vi "SVG2VSDX.vi"() -> ()   [LabVIEW 2018]
uses:
  <userlib>/_OpenG.lib/file/file.llb/Convert File Extension (Path)__ogtk.vi
panel:
  in  "使用源路径":bool=TRUE
  in  "Viso格式":enum32{"VSD", "VSDX"}(radio)=enum."VSDX"
  in  "Viso路径":path
  in  "SVG路径":path
  in  "转换":bool
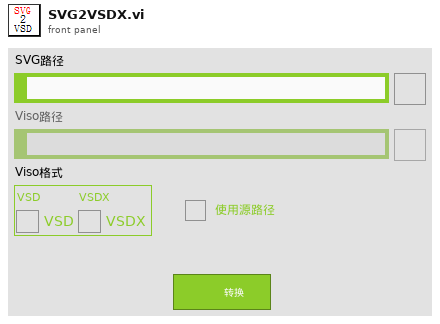
[diagram p1: front panel]
types:
  T1 = enum8{"Enabled", "Disabled", "Disabled and Grayed Out"}
  T2 = enum16{"Null", "NonExist", "EmptyFile", "File", "EmptyDir", "Directory"}
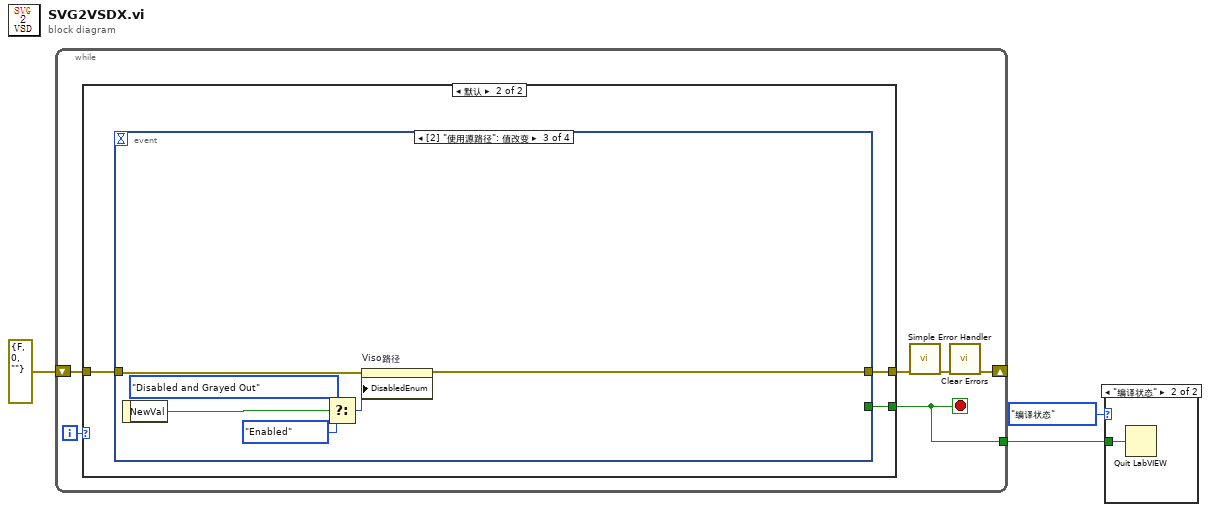
[diagram p0: block diagram]
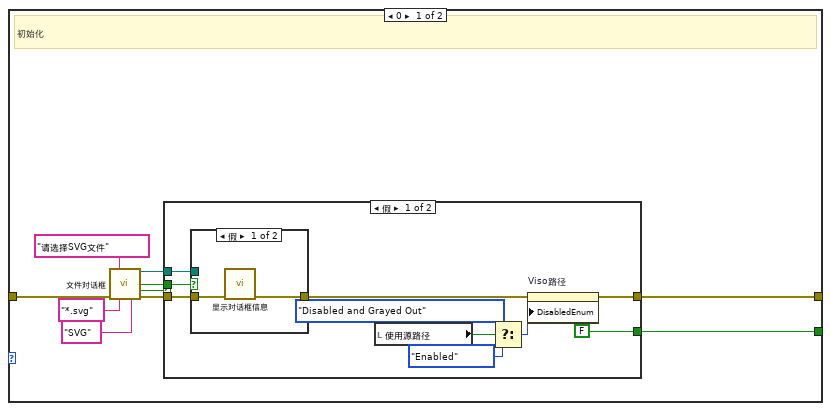
[diagram p3: hidden frame]
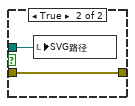
[diagram p4: hidden frame]
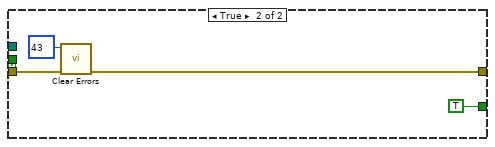
[diagram p5: hidden frame]
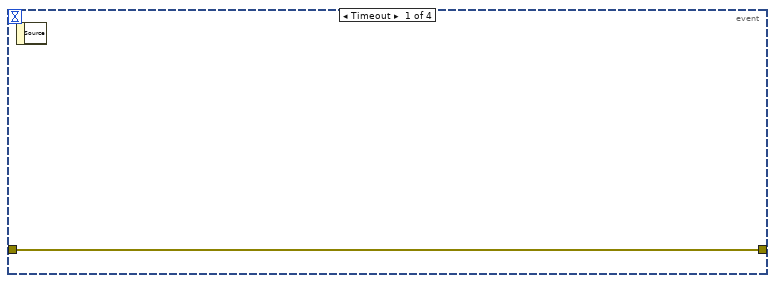
[diagram p6: hidden frame]
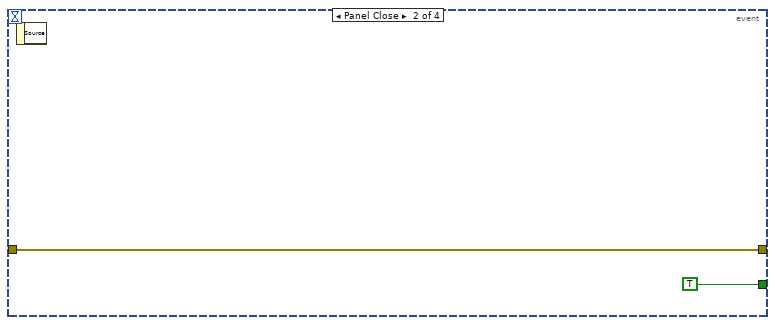
[diagram p7: hidden frame]
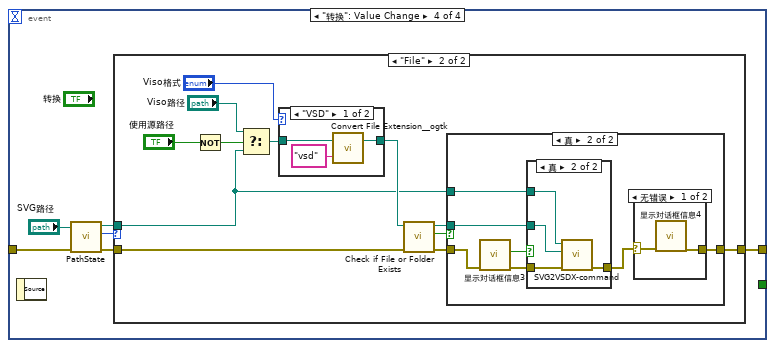
[diagram p8: hidden frame]
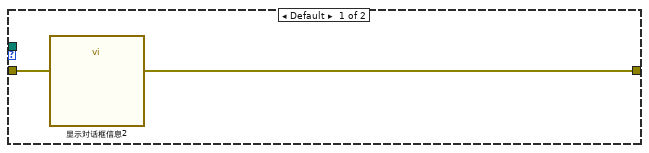
[diagram p9: hidden frame]
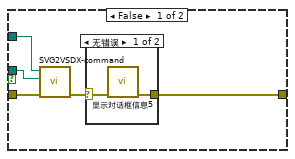
[diagram p10: hidden frame]
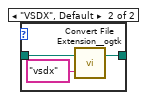
[diagram p14: hidden frame]
diagram:
  n1 = while {
    tunnel: [w4] -> w1
    shift-right: [w5] -> _
    shift-left: errorcluster {"status"=FALSE, "code"=0, "source"=""} ("Error in") -> [w8]
    i -> [w9]
    stop <- w4 stop-if-true
    n2 = case shown="默认" w9 {
      tunnel: w8 -> [w19 w40]
      tunnel: [w10 w39] -> w7
      tunnel: [w13 w38] -> w4
      frame 0 {
        # "初始化"
        n3 = call "文件对话框"("prompt"="请选择SVG文件", "error in"=w19, "pattern (all files)"="*.svg", "pattern label"="SVG") -> ("selected path"=w11:path, "exists"=w12:bool, "cancelled"=w14:bool, "error out"=w18:errorcluster)  [unwired: 8 in]
        n4 = case shown="假" w14 {
          tunnel: w18 -> [w29 w37]
          tunnel: [w25 w36] -> w10
          tunnel: [FALSE TRUE] -> w13
          tunnel: w12 -> [w27 _]
          tunnel: w11 -> [w26 _]
          frame False {
            n5 = case shown="假" w27 {
              tunnel: w29 -> [w31 w33]
              tunnel: [w30 w33] -> w24
              tunnel: w26 -> [_ w32]
              frame False {
                n6 = call "显示对话框信息"("error in (no error)"=w31) -> ("error out"=w30:errorcluster)  [unwired: 9 in, 1 out]
              }
              frame True {
                n7 = local write "SVG路径"(w32) -> ()
              }
            }
            n8 = local read "使用源路径"() -> (w20:bool)
            n9 = Select(t=T1."Disabled and Grayed Out" ("禁用"), s=w20, f=T1."Enabled" ("禁用")) -> (s? t:f=w21:T1)
            n10 = property on="Viso路径" class="Path"(error in=w24, "DisabledEnum"=w21) -> (error out=w25:errorcluster)  [unwired: 1 in, 1 out]
          }
          frame True {
            n11 = call <vilib>:"Clear Errors.vi"("error in (no error)"=w37, "specific error code to clear (0: all)"=43) -> ("error out"=w36:errorcluster)  [unwired: 4 in, 1 out]
          }
        }
      }
      frame Default {
        n12 = event shown="[2] \"使用源路径\": 值改变" {
          selector: _ -> [_ _ _ _]
          dyn-events: _ -> [_ _ _ _]
          timeout: _ -> [_ _ _ _]
          tunnel: w40 -> [w41 w43 w45 w55]
          tunnel: [w41 w43 w46 w52] -> w39
          tunnel: [_ TRUE _ _] -> w38
          event Timeout {
            n13 = event-data() -> ()  [unwired: 1 in, 1 out]
          }
          event Panel Close {
            n14 = event-data() -> ()  [unwired: 1 in, 1 out]
          }
          event "使用源路径": Value Change {
            n15 = event-data() -> ("NewVal"=w44:bool)  [unwired: 1 in]
            n16 = Select(t=T1."Disabled and Grayed Out" ("禁用"), s=w44, f=T1."Enabled" ("禁用")) -> (s? t:f=w47:T1)
            n17 = property on="Viso路径" class="Path"(error in=w45, "DisabledEnum"=w47) -> (error out=w46:errorcluster)  [unwired: 1 in, 1 out]
          }
          event "转换": Value Change {
            n18 = event-data() -> ()  [unwired: 1 in, 1 out]
            n19 = call <vilib>:"PathState.vi"("error in (no error)"=w55, "Path_input"="SVG路径") -> ("error out"=w54:errorcluster, "State"=w51:T2, "Path_output"=w50:path)  [unwired: 7 in]
            n20 = case shown="\"File\"" w51 {
              tunnel: w54 -> [w57 w69]
              tunnel: [w56 w63] -> w52
              tunnel: w50 -> [_ w58]
              frame Default {
                n21 = call "显示对话框信息2"("error in (no error)"=w57) -> ("error out"=w56:errorcluster)  [unwired: 9 in, 1 out]
              }
              frame "File" {
                n22 = Not(x="使用源路径") -> (.not. x?=w66:bool)
                n23 = Select(t="Viso路径", s=w66, f=w58) -> (s? t:f=w64:path)
                n24 = case shown="\"VSD\"" "Viso格式" {
                  tunnel: w64 -> [w95 w98]
                  tunnel: [w93 w96] -> w60
                  frame "VSD" {
                    n25 = call-poly <userlib>:"Convert File Extension__ogtk.vi"("new ending (none)"="vsd", "file name"=w95) -> ("new filename"=w93:path)  [unwired: 1 out]
                  }
                  frame "VSDX", Default {
                    n26 = call-poly <userlib>:"Convert File Extension__ogtk.vi"("new ending (none)"="vsdx", "file name"=w98) -> ("new filename"=w96:path)  [unwired: 1 out]
                  }
                }
                n27 = call <vilib>:"Check if File or Folder Exists.vi"("error in (no error)"=w69, "path"=w60) -> ("error out"=w62:errorcluster, "file or folder exists?"=w61:bool, "dup path"=w59:path)  [unwired: 7 in]
                n28 = case shown="真" w61 {
                  tunnel: w62 -> [w74 w84]
                  tunnel: [w71 w79] -> w63
                  tunnel: w59 -> [w72 w81]
                  tunnel: w58 -> [w73 w80]
                  frame False {
                    n29 = call "SVG2VSDX-command.vi"("Error in"=w74, "vsd路径"=w72, "svg路径"=w73) -> ("Error out"=w70:errorcluster)  [unwired: 8 in]
                    n30 = case shown="无错误" w70 {
                      selector: w70 -> [w75 w77]
                      tunnel: [w76 w77] -> w71
                      frame No Error {
                        n31 = call "显示对话框信息5"("error in (no error)"=w75) -> ("error out"=w76:errorcluster)  [unwired: 9 in, 1 out]
                      }
                      frame Error {
                      }
                    }
                  }
                  frame True {
                    n32 = call "显示对话框信息3"("error in (no error)"=w84) -> ("error out"=w83:errorcluster, "是"=w82:bool)  [unwired: 9 in]
                    n33 = case shown="真" w82 {
                      tunnel: w83 -> [w88 w92]
                      tunnel: [w88 w91] -> w78
                      tunnel: w81 -> [_ w90]
                      tunnel: w80 -> [_ w89]
                      frame False {
                      }
                      frame True {
                        n34 = call "SVG2VSDX-command.vi"("Error in"=w92, "vsd路径"=w90, "svg路径"=w89) -> ("Error out"=w91:errorcluster)  [unwired: 8 in]
                      }
                    }
                    n35 = case shown="无错误" w78 {
                      selector: w78 -> [w85 w87]
                      tunnel: [w86 w87] -> w79
                      frame No Error {
                        n36 = call "显示对话框信息4"("error in (no error)"=w85) -> ("error out"=w86:errorcluster)  [unwired: 9 in, 1 out]
                      }
                      frame Error {
                      }
                    }
                  }
                }
              }
            }
          }
        }
      }
    }
    n37 = call <vilib>:"Simple Error Handler.vi"("error in (no error)"=w7) -> ("error out"=w6:errorcluster)  [unwired: 4 in, 4 out]
    n38 = call <vilib>:"Clear Errors.vi"("error in (no error)"=w6) -> ("error out"=w5:errorcluster)  [unwired: 5 in, 1 out]
  }
  n39 = case shown="\"编译状态\"" enum16{"设计状态", "编译状态"}."编译状态" {
    tunnel: w1 -> [_ w99]
    frame "设计状态", Default {
    }
    frame "编译状态" {
      n40 = Quit LabVIEW(quit? (T)=w99) -> ()
    }
  }
